vi "control_to_register.vi"(11 "config_channels":T2[](array[typedef])) -> (3 "Channels":T1(array[cluster]))   [LabVIEW 2016]
uses:
  config_board.ctl
panel:
  in  "Acelerômetro":T3
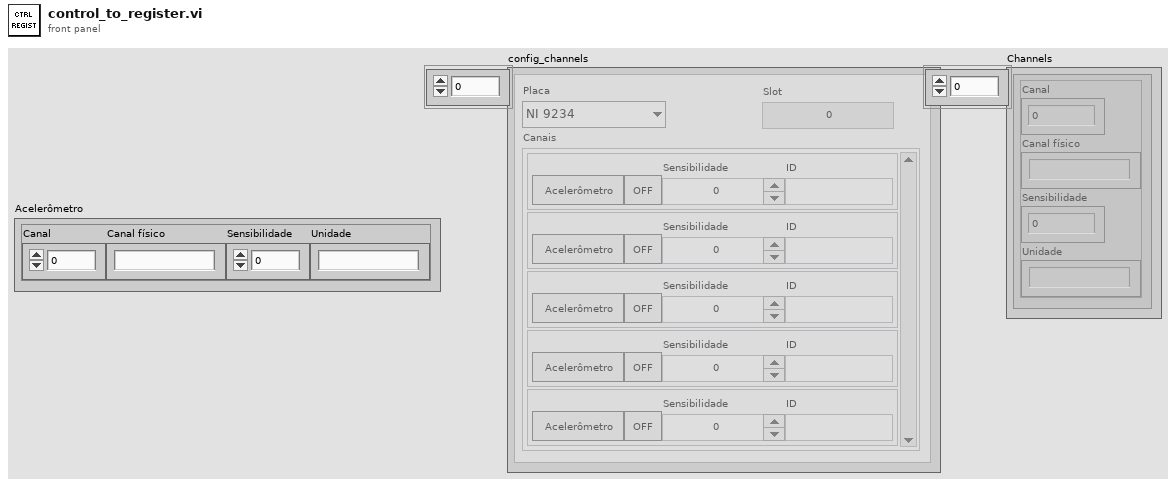
[diagram p1: front panel]
types:
  T1 = cluster{"Canal":i32, "Canal físico":string, "Sensibilidade":dbl, "Unidade":string}[]
  T2 = typedef "config_board.ctl" = cluster{"board":enum16{"NI 9234", "NI 9205", "Não aplicável"}, "channels":cluster{"type":bool, "active":bool, "sens":dbl, "ID":string}[], "Slot":i32}
  T3 = cluster{"Canal":i32, "Canal físico":string, "Sensibilidade":dbl, "Unidade":string}
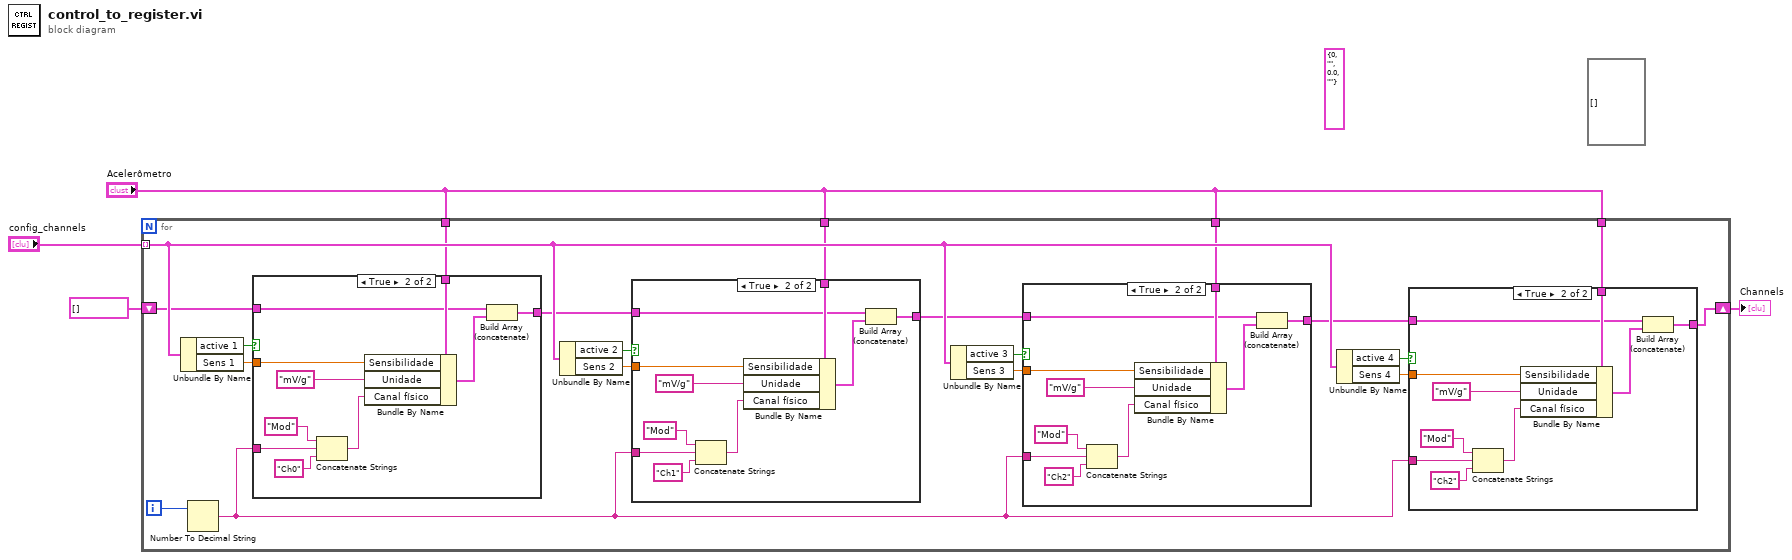
[diagram p0: block diagram]
diagram:
  (unwired) T3 {"Canal"=0, "Canal físico"="", "Sensibilidade"=0.0, "Unidade"=""} ("Acelerômetro")
  (unwired) void[] [] ("Channels 2")
  n1 = for {
    tunnel: "config_channels" -> [w24] mode=indexing
    tunnel: "Acelerômetro" -> [w23]
    shift-right: [w6] -> w1
    shift-left: T1 [] -> [w19]
    tunnel: "Acelerômetro" -> [w15]
    tunnel: "Acelerômetro" -> [w11]
    tunnel: "Acelerômetro" -> [w7]
    i -> [w20]
    n2 = Unbundle By Name(w24) -> ("active 1"=w22:bool, "Sens 1"=w21:dbl)
    n3 = Number To Decimal String(number=w20) -> (decimal integer string=w5:string)  [unwired: 1 in]
    n4 = case shown="True" w22 {
      tunnel: w23 -> [_ w57]
      tunnel: w21 -> [_ w56]
      tunnel: w5 -> [_ w53]
      tunnel: [w47 w49] -> w16
      tunnel: w19 -> [w47 w48]
      frame False {
      }
      frame True {
        n5 = Concatenate Strings("Mod" ("string"), w53, "Ch0" ("string")) -> (w51:string)
        n6 = Bundle By Name(cluster=w57, "Sensibilidade"=w56, "Unidade"="mV/g", "Canal físico"=w51) -> (w50:T3)
        n7 = Build Array (concatenate)(w48, w50) -> (w49:T1)
      }
    }
    n8 = Unbundle By Name(w24) -> ("active 2"=w17:bool, "Sens 2"=w18:dbl)
    n9 = case shown="True" w17 {
      tunnel: w15 -> [_ w46]
      tunnel: w18 -> [_ w45]
      tunnel: w5 -> [_ w42]
      tunnel: [w36 w38] -> w12
      tunnel: w16 -> [w36 w37]
      frame False {
      }
      frame True {
        n10 = Concatenate Strings("Mod" ("string"), w42, "Ch1" ("string")) -> (w40:string)
        n11 = Bundle By Name(cluster=w46, "Sensibilidade"=w45, "Unidade"="mV/g", "Canal físico"=w40) -> (w39:T3)
        n12 = Build Array (concatenate)(w37, w39) -> (w38:T1)
      }
    }
    n13 = Unbundle By Name(w24) -> ("active 3"=w14:bool, "Sens 3"=w13:dbl)
    n14 = case shown="True" w14 {
      tunnel: w11 -> [_ w35]
      tunnel: w13 -> [_ w34]
      tunnel: w5 -> [_ w31]
      tunnel: [w25 w27] -> w8
      tunnel: w12 -> [w25 w26]
      frame False {
      }
      frame True {
        n15 = Concatenate Strings("Mod" ("string"), w31, "Ch2" ("string")) -> (w29:string)
        n16 = Bundle By Name(cluster=w35, "Sensibilidade"=w34, "Unidade"="mV/g", "Canal físico"=w29) -> (w28:T3)
        n17 = Build Array (concatenate)(w26, w28) -> (w27:T1)
      }
    }
    n18 = Unbundle By Name(w24) -> ("active 4"=w9:bool, "Sens 4"=w10:dbl)
    n19 = case shown="True" w9 {
      tunnel: w7 -> [_ w68]
      tunnel: w10 -> [_ w67]
      tunnel: w5 -> [_ w64]
      tunnel: [w58 w60] -> w6
      tunnel: w8 -> [w58 w59]
      frame False {
      }
      frame True {
        n20 = Concatenate Strings("Mod" ("string"), w64, "Ch2" ("string")) -> (w62:string)
        n21 = Bundle By Name(cluster=w68, "Sensibilidade"=w67, "Unidade"="mV/g", "Canal físico"=w62) -> (w61:T3)
        n22 = Build Array (concatenate)(w59, w61) -> (w60:T1)
      }
    }
  }
  "Channels" <- w1
